vi "RMGetBeadResults.vi"(7 "bead":i32, 8 "error in (no error)":errorcluster, 9 "numFrames":i32, 10 "startFrame (0)":i32, 11 "ResultManager":T4={"InstancePtr"=0, "ResultManagerConfig"={"Number of beads"=0, "Number of frame info columns"=0, "Result scaling"={"X"=0.0, "Y"=0.0, "Z"=0.0}, "Result offset"={"X"=0.0, "Y"=0.0, "Z"=0.0}, "Write Interval"=100, "Max frames in memory"=100, "Binary output (1/0)"=0}}) -> (0 "error out":errorcluster, 2 "results":T1[](array[typedef]), 3 "ResultManager (out)":T4={"InstancePtr"=0, "ResultManagerConfig"={"Number of beads"=0, "Number of frame info columns"=0, "Result scaling"={"X"=0.0, "Y"=0.0, "Z"=0.0}, "Result offset"={"X"=0.0, "Y"=0.0, "Z"=0.0}, "Write Interval"=100, "Max frames in memory"=100, "Binary output (1/0)"=0}})   [LabVIEW 2011]
uses:
  ResultManagerInstance.ctl
  ResultManagerConfig.ctl
  XYZf.ctl
  QTrkLocalizationResult.ctl
  QTrkLocalizationJob.ctl
  QTrkDLL.vi
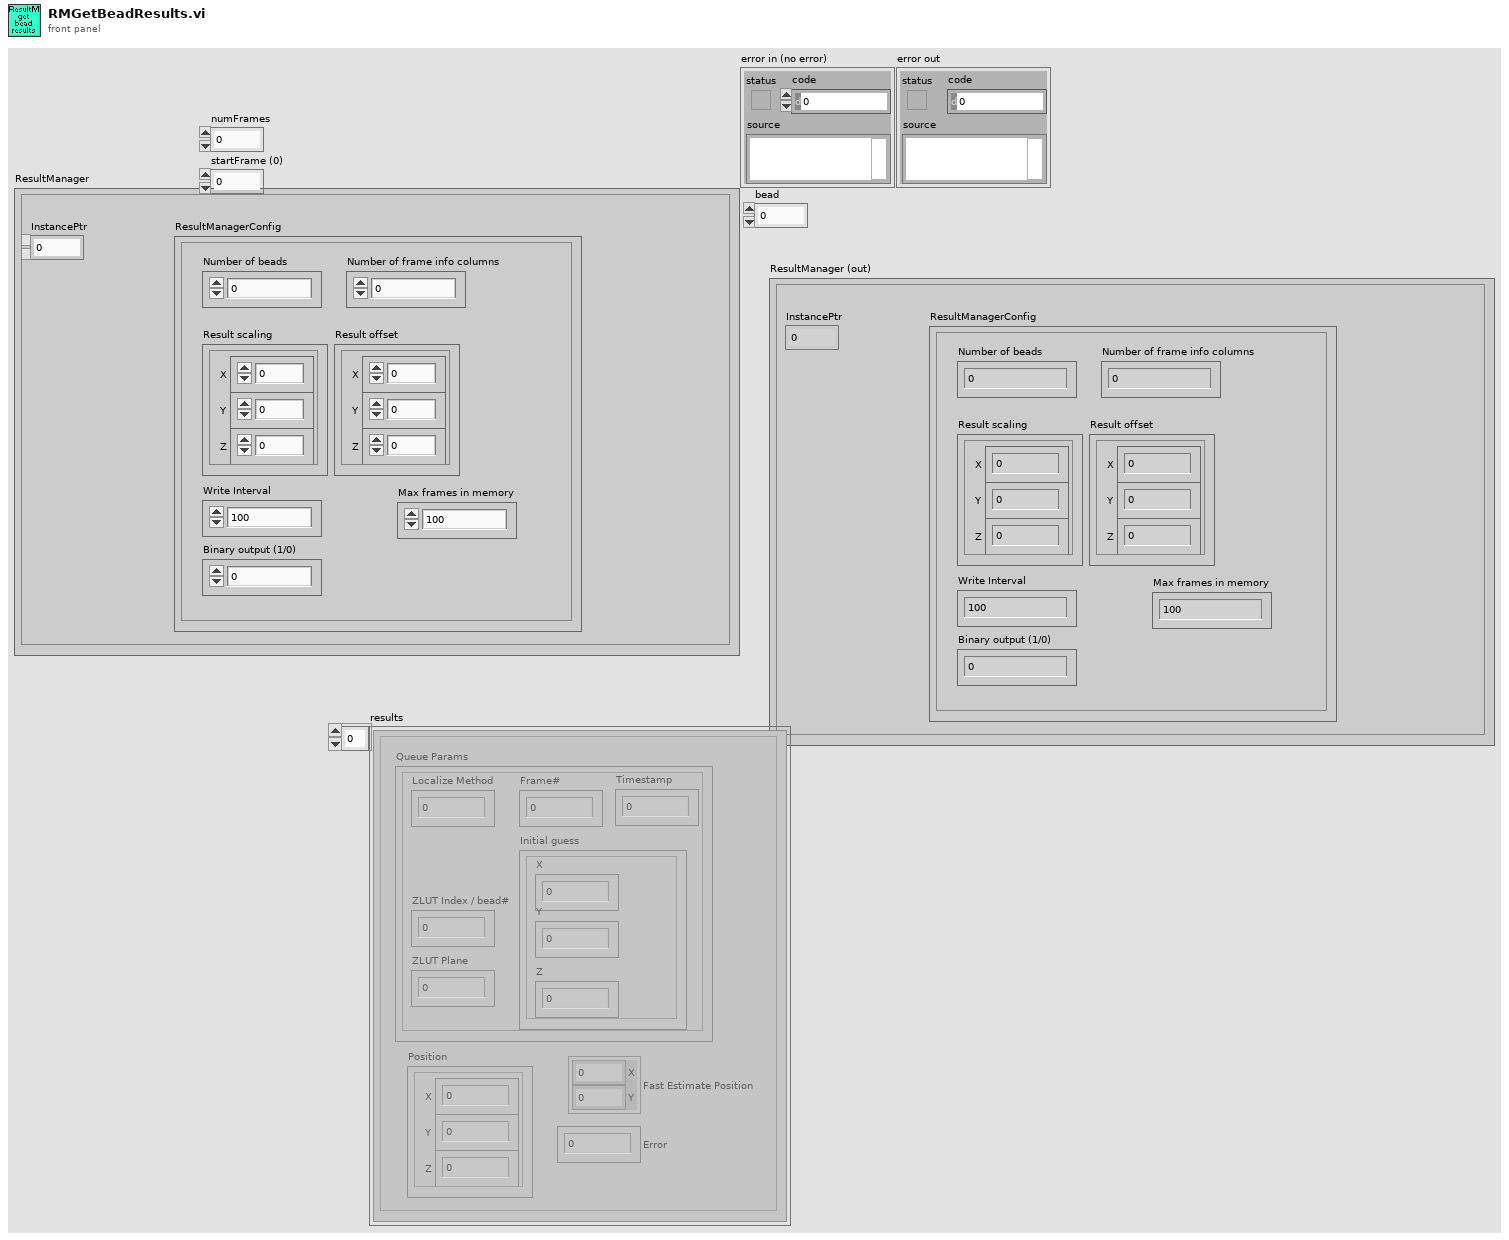
[diagram p1: front panel]
types:
  T1 = typedef "QTrkLocalizationResult.ctl" = cluster{"Queue Params":T2, "Position":T3, "Fast Estimate Position":cluster{"X":sgl, "Y":sgl}, "Error":i32}
  T2 = typedef "QTrkLocalizationJob.ctl" = cluster{"Localize Method":i32, "Frame#":u32, "Timestamp":u32, "ZLUT Index / bead#":i32, "ZLUT Plane":i32, "Initial guess":T3}
  T3 = typedef "XYZf.ctl" = cluster{"X":sgl, "Y":sgl, "Z":sgl}
  T4 = typedef "ResultManagerInstance.ctl" = cluster{"InstancePtr":u64, "ResultManagerConfig":T5}
  T5 = typedef "ResultManagerConfig.ctl" = cluster{"Number of beads":i32, "Number of frame info columns":i32, "Result scaling":T3, "Result offset":T3, "Write Interval":i32, "Max frames in memory":i32, "Binary output (1/0)":i8}
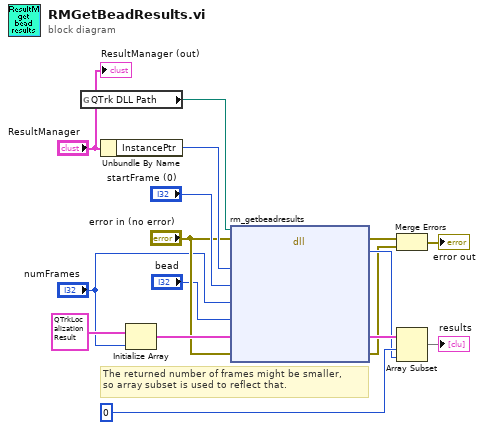
[diagram p0: block diagram]
diagram:
  # "The returned number of frames might be smaller, \nso array subset is used to reflect that."
  n1 = global read "QTrkDLL.vi" "QTrk DLL Path"() -> (w16:path)
  n2 = Unbundle By Name("ResultManager") -> ("InstancePtr"=w7:u64)
  n3 = Initialize Array(T1 {"Queue Params"={"Localize Method"=0, "Frame#"=0, "Timestamp"=0, "ZLUT Index / bead#"=0, "ZLUT Plane"=0, "Initial guess"={"X"=0.0, "Y"=0.0, "Z"=0.0}}, "Position"={"X"=0.0, "Y"=0.0, "Z"=0.0}, "Fast Estimate Position"={"X"=0.0, "Y"=0.0}, "Error"=0} ("Localization Result"), "numFrames") -> (w14:T1[])
  n4 = dll-call lib="D:/labview/jelmer/version ctrl/bin/jtrk-labview.dll" fn="rm_getbeadresults"(path in=w16, error in="error in (no error)", "resultmanager"=w7, "startFrame"="startFrame (0)", "numFrames"="numFrames", "bead"="bead", "results"=w14, "error"="error in (no error)") -> (error out=w5:errorcluster, "result count"=w10:i32, "results"=w12:T1[], "error"=w4:errorcluster)  [unwired: 5 in, 1 out]
  n5 = Merge Errors(w5, w4) -> (→"error out":errorcluster)
  n6 = Array Subset(array=w12, index=0, length=w10) -> (→"results":T1[])
  "ResultManager (out)" <- "ResultManager"
